vi "ryTimer Get Properties.vi"(8 "error in (no error)":errorcluster, 11 "ryTimer in":refnum<class "ryTimer.lvclass">) -> (0 "error out":errorcluster, 2 "Properties":refnum<data-value>, 3 "ryTimer out":refnum<class "ryTimer.lvclass">)   [LabVIEW 2020, in "ryTimer.lvclass"]
uses:
  ryTimer.lvclass
  TypeDefs/ryTimer Properties.ctl
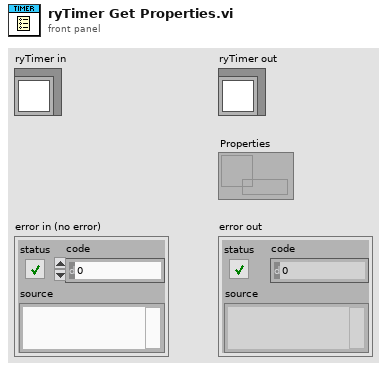
[diagram p1: front panel]
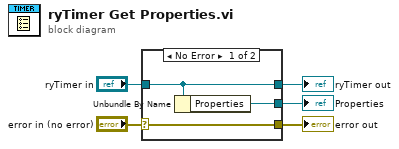
[diagram p0: block diagram]
diagram:
  n1 = case shown="No Error" "error in (no error)" {
    selector: "error in (no error)" -> [w8 w9]
    tunnel: [w8 w9] -> w4
    tunnel: [w7 w10] -> w2
    tunnel: "ryTimer in" -> [w7 w10]
    tunnel: [w6 _] -> w1
    frame No Error {
      n2 = Unbundle By Name(w7) -> ("Properties"=w6:refnum<data-value>)
    }
    frame Error {
    }
  }
  "error out" <- w4
  "ryTimer out" <- w2
  "Properties" <- w1
